vi "EMD8216 security unlock.vi"(10 "password":string, 11 "CardID":u32) -> (3 "error_code":u32)   [LabVIEW 2015, in "EMD8216_64.lvlib"]
doc: "EMD8216Status EMD8216_security_unlock(u32 CardID,u8 password[8]);"
uses:
  EMD8216_64.lvlib
  EMD8216_64.dll
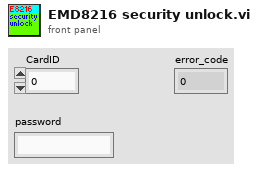
[diagram p1: front panel]
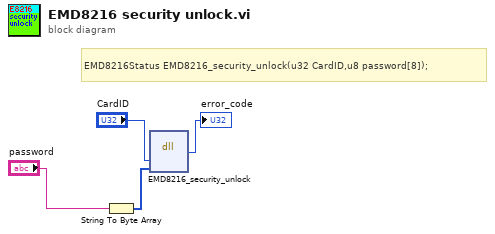
[diagram p0: block diagram]
diagram:
  # "EMD8216Status EMD8216_security_unlock(u32 CardID,u8 password[8]);"
  n1 = String To Byte Array(string="password") -> (unsigned byte array=w1:u8[])
  n2 = dll-call lib="C:/Users/jeff.lin.MINAIK/Documents/Soulkai/Labview/io/EMD8216_64/EMD8216_64/EMD8216_64.*" fn="EMD8216_security_unlock"("CardID"="CardID", "password"=w1) -> ("return type"=→"error_code":u32)  [unwired: 5 in, 2 out]
